vi "Acquire.vi"(5 "Initial Y Conditions":dbl[][](array[numeric]), 7 "Initial X Conditions":dbl[][](array[numeric]), 8 "error in (no error)":errorcluster, 9 "Data Queue":refnum<queue>, 10 "Data Notifier":refnum<notifier>, 11 "Hardware Resources in":T1={"DAQmx Channel"="cDAQETH/ai0:23, cDAQETH/ai29, cDAQETH/ai31:30", "Sample Rate"=0.0, "DAQmx Task"="", "ResetInterp"=TRUE, "GainConstants"=[0.01, 0.2, 10.0, 1.0, 0.1], "FilterCoefficients"=[], "ChannelNames"=[], "ActiveChannels"=[], "Display Rate"=1000, "ResponseExtension"=TRUE}) -> (0 "error out":errorcluster, 3 "Hardware Resources out":T1={"DAQmx Channel"="", "Sample Rate"=0.0, "DAQmx Task"="", "ResetInterp"=FALSE, "GainConstants"=[], "FilterCoefficients"=[], "ChannelNames"=[], "ActiveChannels"=[], "Display Rate"=1000, "ResponseExtension"=TRUE}, 4 "Final Y Conditions":dbl[][](array[numeric]), 6 "Final X Conditions":dbl[][](array[numeric]))   [LabVIEW 2017, in "Acquisition.lvlib"]
doc: "Perform the acquisition. Replace the contents of this diagram with calls to acquisition hardware."
uses:
  Acquisition.lvlib
  Hardware Configuration.ctl
  <vilib>/DAQmx/read.llb/DAQmx Read (Analog 1D Wfm NChan NSamp).vi
  <vilib>/Analysis/baseanly.llb/Mean (DBL).vi
  <vilib>/Analysis/3filter.llb/IIR Filter with I.C. (DBL).vi
  <vilib>/DAQmx/miscellaneous.llb/DAQmx Fill In Error Info.vi
  <vilib>/measure/maresamp.llb/Align N Waveforms (continuous).vi
  <vilib>/measure/maresamp.llb/Resample N Waveforms (continuous).vi
  <resource>/objmgr/daqmx.rc
  <vilib>/measure/NI_MAPro.lvlib
  <vilib>/Analysis/NI_AALBase.lvlib
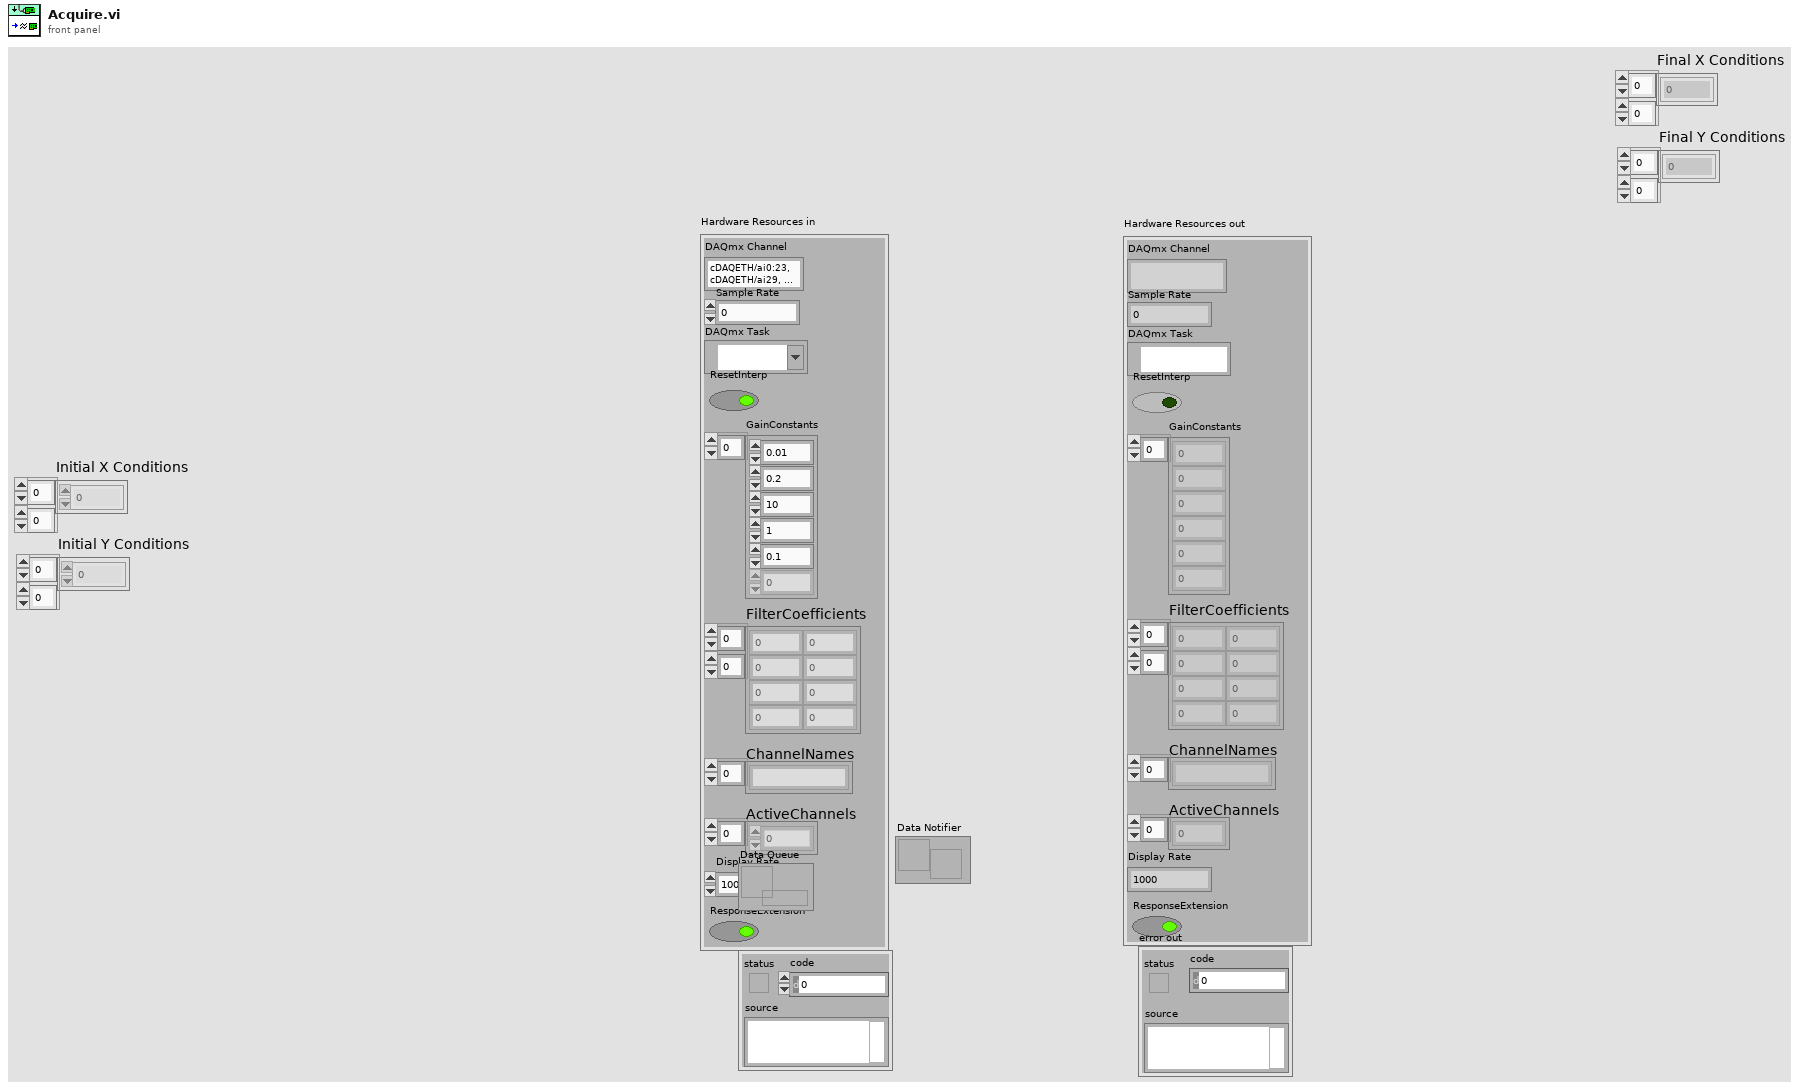
[diagram p1: front panel]
types:
  T1 = typedef "Acquisition.lvlib/Hardware Configuration.ctl" = cluster{"DAQmx Channel":string, "Sample Rate":dbl, "DAQmx Task":refnum<k21>, "ResetInterp":bool, "GainConstants":dbl[], "FilterCoefficients":dbl[][], "ChannelNames":string[], "ActiveChannels":i32[], "Display Rate":i32, "ResponseExtension":bool}
  T2 = cluster{"alias rejection (dB)":dbl, "normalized bandwidth":dbl}
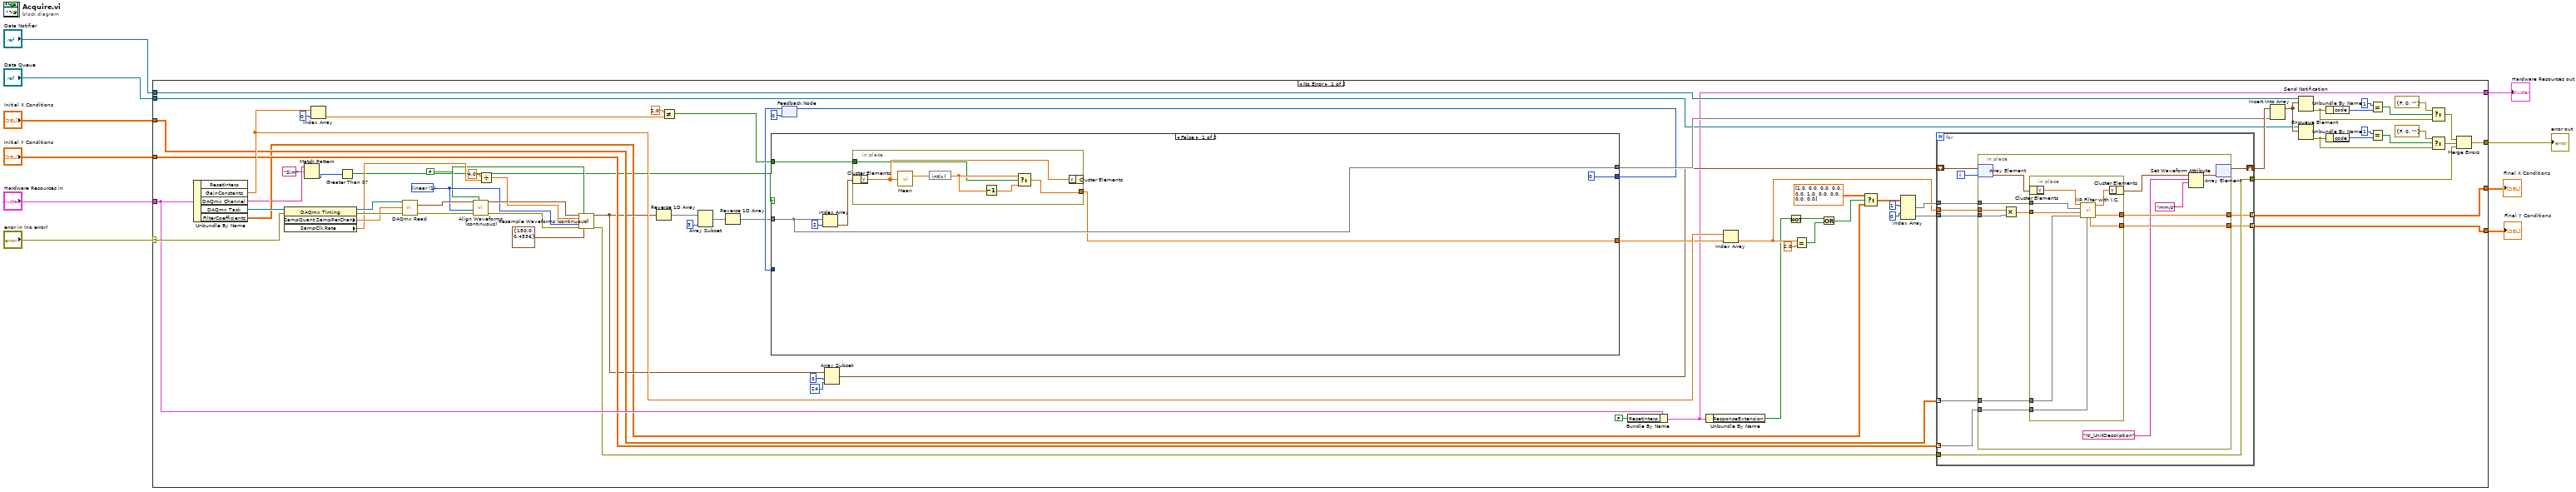
[diagram p0: block diagram]
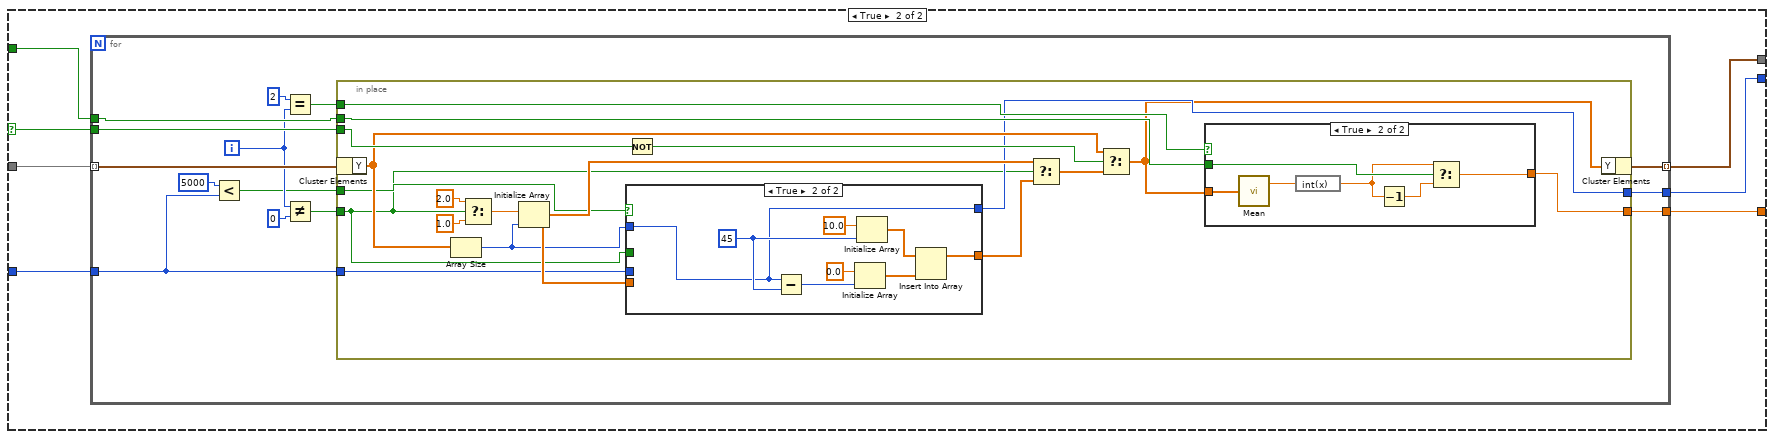
[diagram p2: hidden frame]
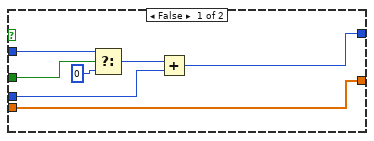
[diagram p3: hidden frame]
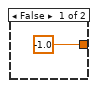
[diagram p4: hidden frame]
diagram:
  n1 = case shown="No Error" "error in (no error)" {
    selector: "error in (no error)" -> [w74 w194]
    tunnel: [w86 w194] -> w9
    tunnel: "Hardware Resources in" -> [w68 w195]
    tunnel: [w17 w195] -> w7
    tunnel: "Data Notifier" -> [w27 _]
    tunnel: "Data Queue" -> [w26 _]
    tunnel: [w58 w192] -> w4
    tunnel: [w57 w193] -> w3
    tunnel: "Initial X Conditions" -> [w56 w193]
    tunnel: "Initial Y Conditions" -> [w55 w192]
    frame No Error {
      w25 = FALSE ("reset")
      w45 = u16 1 items=["coerce", "linear", "spline", "FIR filter"] ("interpolation mode")
      n2 = Unbundle By Name(w68) -> ("GainConstants"=w59:dbl[], "DAQmx Channel"=w14:string, "DAQmx Task"=w69:refnum<k21>, "FilterCoefficients"=w20:dbl[][])  [unwired: 1 out]
      n3 = property class="DAQmx Timing"(reference=w69, error in=w74) -> (reference out=w75:refnum<k21>, error out=w73:errorcluster, "SampQuant.SampPerChan"=w63:dbl, "SampClk.Rate"=w61:dbl)
      n4 = Match Pattern(string=w14, regular expression="Sim") -> (offset past match=w12:i32)  [unwired: 1 in, 3 out]
      n5 = Index Array(array=w59, index=0) -> (element=w47:dbl)
      n6 = Greater Than 0?(x=w12) -> (x > 0?=w11:bool)
      n7 = call-poly <vilib>:"DAQmx Read.vi"("task/channels in"=w75, "number of samples per channel"=w63, "error in"=w73) -> ("data"=w70:waveform(dbl)[], "error out"=w71:errorcluster)  [unwired: 10 in, 1 out]
      n8 = call-poly <vilib>:"Align Waveforms (continuous).vi"("reset"=w25, "error in (no error)"=w71, "interpolation mode"=w45, "waveforms in"=w70) -> ("error out"=w49:errorcluster, "waveforms out"=w50:waveform(dbl)[])  [unwired: 6 in]
      n9 = Divide(x=4.0, y=w61) -> (x/y=w60:dbl)
      n10 = call-poly <vilib>:"Resample Waveforms (continuous).vi"("waveforms in"=w50, "reset"=w25, "dt"=w60, "interpolation mode"=w45, "error in (no error)"=w49, "FIR filter specifications"=T2 {"alias rejection (dB)"=150.0, "normalized bandwidth"=0.4536}) -> ("resampled waveforms out"=w37:waveform(dbl)[], "error out"=w51:errorcluster)  [unwired: 5 in, 3 out]
      n11 = Reverse 1D Array(array=w37) -> (reversed array=w34:waveform(dbl)[])
      n12 = Not Equal?(x=2.0, y=w47) -> (x != y?=w42:bool)
      n13 = Array Subset(array=w34, length=3) -> (w36:waveform(dbl)[])  [unwired: 1 in]
      n14 = Reverse 1D Array(array=w36) -> (reversed array=w35:waveform(dbl)[])
      n15 = feedback #1(0) -> (w40:i32)
      n16 = case shown="False" w11 {
        selector: w11 -> [_ w99]
        tunnel: [w92 w105] -> w44
        tunnel: w42 -> [w89 w104]
        tunnel: [w88 w103] -> w41
        tunnel: w40 -> [_ w102]
        tunnel: [0 w101] -> w39
        tunnel: w35 -> [w92 w100]
        frame False {
          n17 = Index Array(array=w92, index=2) -> (element=w90:waveform(dbl))
          n18 = in-place {
            in-place-border: [w98] -> w88
            in-place-border: w89 -> [w93]
            n19 = in-place-cluster #2(w90) -> ("Y"=w97:dbl[])
            n20 = call-poly <vilib>:"Mean.vi"("X"=w97) -> ("mean"=w96:dbl)  [unwired: 1 out]
            n21 = expression code="int(x)"(w96) -> (w95:dbl)
            n22 = Decrement(x=w95) -> (x-1=w94:dbl)
            n23 = Select(t=w95, s=w93, f=w94) -> (s? t:f=w98:dbl)
            n24 = in-place-cluster #2("Y"=w97) -> ()  [unwired: 1 out]
          }
        }
        frame True {
          n25 = for {
            tunnel: w100 -> [w119] mode=indexing
            tunnel: [w118] -> w105 mode=indexing
            tunnel: w99 -> [w117]
            tunnel: w104 -> [w116]
            tunnel: [w115] -> w103
            tunnel: w102 -> [w107]
            tunnel: [w109] -> w101
            i -> [w111]
            n26 = Less?(x=5000, y=w107) -> (x < y?=w108:bool)
            n27 = Equal?(x=2 ("y"), y=w111) -> (x = y?=w114:bool)
            n28 = Not Equal?(x=w111, y=0) -> (x != y?=w110:bool)
            n29 = in-place {
              in-place-border: w117 -> [w137]
              in-place-border: w116 -> [w135]
              in-place-border: [w134] -> w115
              in-place-border: w114 -> [w131]
              in-place-border: w110 -> [w121]
              in-place-border: w107 -> [w123]
              in-place-border: [w124] -> w109
              in-place-border: w108 -> [w122]
              n30 = in-place-cluster #3(w119) -> ("Y"=w132:dbl[])
              n31 = Array Size(array=w132) -> (size(s)=w125:i32)
              n32 = Select(t=2.0, s=w121, f=1.0 ("element")) -> (s? t:f=w127:dbl)
              n33 = Initialize Array(w127, w125) -> (w129:dbl[])
              n34 = case shown="True" w122 {
                tunnel: w129 -> [w144 _]
                tunnel: [w144 w145] -> w128
                tunnel: w125 -> [w139 w149]
                tunnel: [w143 w149] -> w124
                tunnel: w123 -> [w142 _]
                tunnel: w121 -> [w140 _]
                frame False {
                  n35 = Select(t=w139, s=w140, f=0) -> (s? t:f=w141:i32)
                  n36 = Add(x=w141, y=w142) -> (x+y=w143:i32)
                }
                frame True {
                  w150 = 45
                  n37 = Subtract(x=w149, y=w150) -> (x-y=w151:i32)
                  n38 = Initialize Array(0.0 ("element"), w151) -> (w146:dbl[])
                  n39 = Initialize Array(10.0 ("element"), w150) -> (w147:dbl[])
                  n40 = Insert Into Array(array=w147, new element=w146) -> (w145:dbl[])  [unwired: 1 in]
                }
              }
              n41 = Not(x=w137) -> (.not. x?=w133:bool)
              n42 = Select(t=w129, s=w121, f=w128) -> (s? t:f=w130:dbl[])
              n43 = Select(t=w132, s=w133, f=w130) -> (s? t:f=w120:dbl[])
              n44 = case shown="True" w131 {
                tunnel: w135 -> [_ w158]
                tunnel: [-1.0 ("mean") w157] -> w134
                tunnel: w120 -> [_ w156]
                frame False {
                }
                frame True {
                  n45 = call-poly <vilib>:"Mean.vi"("X"=w156) -> ("mean"=w159:dbl)  [unwired: 1 out]
                  n46 = expression code="int(x)"(w159) -> (w155:dbl)
                  n47 = Decrement(x=w155) -> (x-1=w154:dbl)
                  n48 = Select(t=w155, s=w158, f=w154) -> (s? t:f=w157:dbl)
                }
              }
              n49 = in-place-cluster #3("Y"=w120) -> (w118:waveform(dbl))
            }
          }
        }
      }
      n50 = feedback-in #1(w39) -> ()
      n51 = Array Subset(array=w37, index=0, length=24) -> (w28:waveform(dbl)[])
      n52 = Bundle By Name(cluster=w68, "ResetInterp"=FALSE) -> (w17:T1)
      n53 = Unbundle By Name(w17) -> ("ResponseExtension"=w16:bool)
      n54 = Index Array(array=w59, index=w41) -> (element=w24:dbl)
      n55 = Not(x=w16) -> (.not. x?=w15:bool)
      n56 = Equal?(x=w24, y=2.0) -> (x = y?=w22:bool)
      n57 = Or(x=w15, y=w22) -> (x .or. y?=w18:bool)
      n58 = Select(t=dbl[][] [[1.0, 0.0, 0.0, 0.0, 0.0], [1.0, 0.0, 0.0, 0.0, 0.0]] ("FilterCoefficients"), s=w18, f=w20) -> (s? t:f=w19:dbl[][])
      n59 = Index Array(array=w19, index (row) #1=1 ("index (row)"), index (row) #2=0 ("index (row)")) -> (element #1=w30:dbl[], element #2=w29:dbl[])  [unwired: 2 in]
      n60 = for {
        tunnel: w24 -> [w160]
        tunnel: w51 -> [w170]
        tunnel: [w170] -> w66
        tunnel: w29 -> [w169]
        tunnel: w30 -> [w168]
        tunnel: w56 -> [w167] mode=indexing
        tunnel: w55 -> [w166] mode=indexing
        tunnel: [w165] -> w58 mode=indexing
        tunnel: [w164] -> w57 mode=indexing
        shift-right: [w162] -> w54
        shift-left: w28 -> [w161]
        i -> [w163]
        n61 = in-place {
          in-place-border: w169 -> [w183]
          in-place-border: w168 -> [w173]
          in-place-border: w167 -> [w182]
          in-place-border: w166 -> [w181]
          in-place-border: [w180] -> w165
          in-place-border: [w179] -> w164
          in-place-border: w160 -> [w171]
          n62 = in-place-array #4(w161, w163) -> (w178:waveform(dbl))
          n63 = Multiply(x=w171, y=w183) -> (x*y=w172:dbl[])
          n64 = in-place {
            in-place-border: w172 -> [w189]
            in-place-border: w173 -> [w188]
            in-place-border: w182 -> [w185]
            in-place-border: w181 -> [w184]
            in-place-border: [w187] -> w180
            in-place-border: [w186] -> w179
            n65 = in-place-cluster #5(w178) -> ("Y"=w190:dbl[])
            n66 = call-poly <vilib>:"IIR Filter with I.C..vi"("Initial Y Conditions"=w184, "Initial X Conditions"=w185, "Forward Coefficients"=w189, "Reverse Coefficients"=w188, "X"=w190) -> ("Final X Conditions"=w186:dbl[], "Final Y Conditions"=w187:dbl[], "Filtered X"=w191:dbl[])  [unwired: 2 in, 1 out]
            n67 = in-place-cluster #5("Y"=w191) -> (w177:waveform(dbl))
          }
          n68 = Set Waveform Attribute(5:"mm/s" ("name"), 6:"NI_UnitDescription" ("name"), 7:w177) -> (3:w176:waveform(dbl))  [unwired: 1 in, 2 out]
          n69 = in-place-array #4(w176) -> (w162:waveform(dbl)[])  [unwired: 1 out]
        }
      }
      n70 = Insert Into Array(array=w54, new element=w44) -> (w72:waveform(dbl)[])  [unwired: 1 in]
      n71 = Send Notification(notification=w72, notifier=w27) -> (error out=w82:errorcluster)  [unwired: 1 in, 1 out]
      n72 = Enqueue Element(queue=w26, element=w72) -> (error out=w79:errorcluster)  [unwired: 2 in, 2 out]
      n73 = Unbundle By Name(w82) -> ("code"=w85:i32)
      n74 = Unbundle By Name(w79) -> ("code"=w76:i32)
      n75 = Equal?(x=1, y=w85) -> (x = y?=w83:bool)
      n76 = Equal?(x=1, y=w76) -> (x = y?=w78:bool)
      n77 = Select(t=errorcluster {"status"=FALSE, "code"=0, "source"=""} ("error constant"), s=w83, f=w82) -> (s? t:f=w64:errorcluster)
      n78 = Select(t=errorcluster {"status"=FALSE, "code"=0, "source"=""} ("error constant"), s=w78, f=w79) -> (s? t:f=w65:errorcluster)
      n79 = Merge Errors(w64, w65, w66) -> (w86:errorcluster)
    }
    frame Error {
    }
  }
  "Hardware Resources out" <- w7
  "error out" <- w9
  "Final X Conditions" <- w3
  "Final Y Conditions" <- w4
